vi "can开关切换.vi"(8 "输入切换ID":u8, 11 "输出切换ID":u8) -> (2 "成功？":bool)   [LabVIEW 2010]
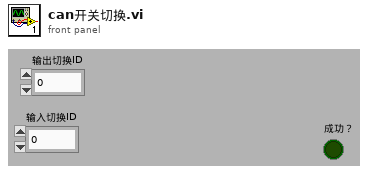
[diagram p1: front panel]
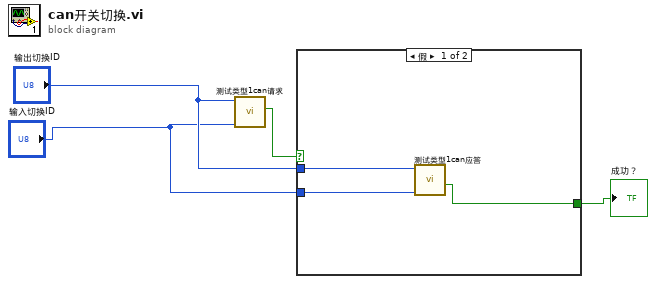
[diagram p0: block diagram]
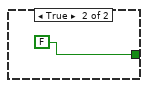
[diagram p2: hidden frame]
diagram:
  n1 = call "测试类型1can请求.vi"("输入切换ID"="输入切换ID", "输出切换ID"="输出切换ID") -> ("发送成功?"=w1:bool)  [unwired: 7 in]
  n2 = case shown="假" w1 {
    tunnel: [w7 FALSE] -> w4
    tunnel: "输出切换ID" -> [w6 _]
    tunnel: "输入切换ID" -> [w5 _]
    frame False {
      n3 = call "测试类型1can应答.vi"("输入切换ID"=w5, "输出切换ID"=w6) -> ("成功？"=w7:bool)  [unwired: 9 in]
    }
    frame True {
    }
  }
  "成功？" <- w4
